vi "SUB_FINDUSB_SND_ID.vi"() -> (3 "Total Sound cards":i32, 4 "PC Sound Card ID":i32, 5 "USB Sound Card ID":i32, 6 "Found USB Snd card":bool)   [LabVIEW 2011]
panel:
  out "Capabilities":T1
  out "Number of Output Devices":i32
  out "Array":string[](array[string])
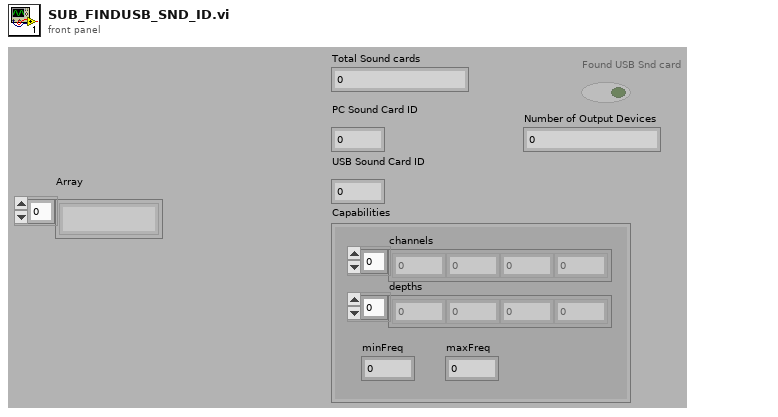
[diagram p1: front panel]
types:
  T1 = cluster{"channels":i32[], "depths":i32[], "minFreq":dbl, "maxFreq":dbl}
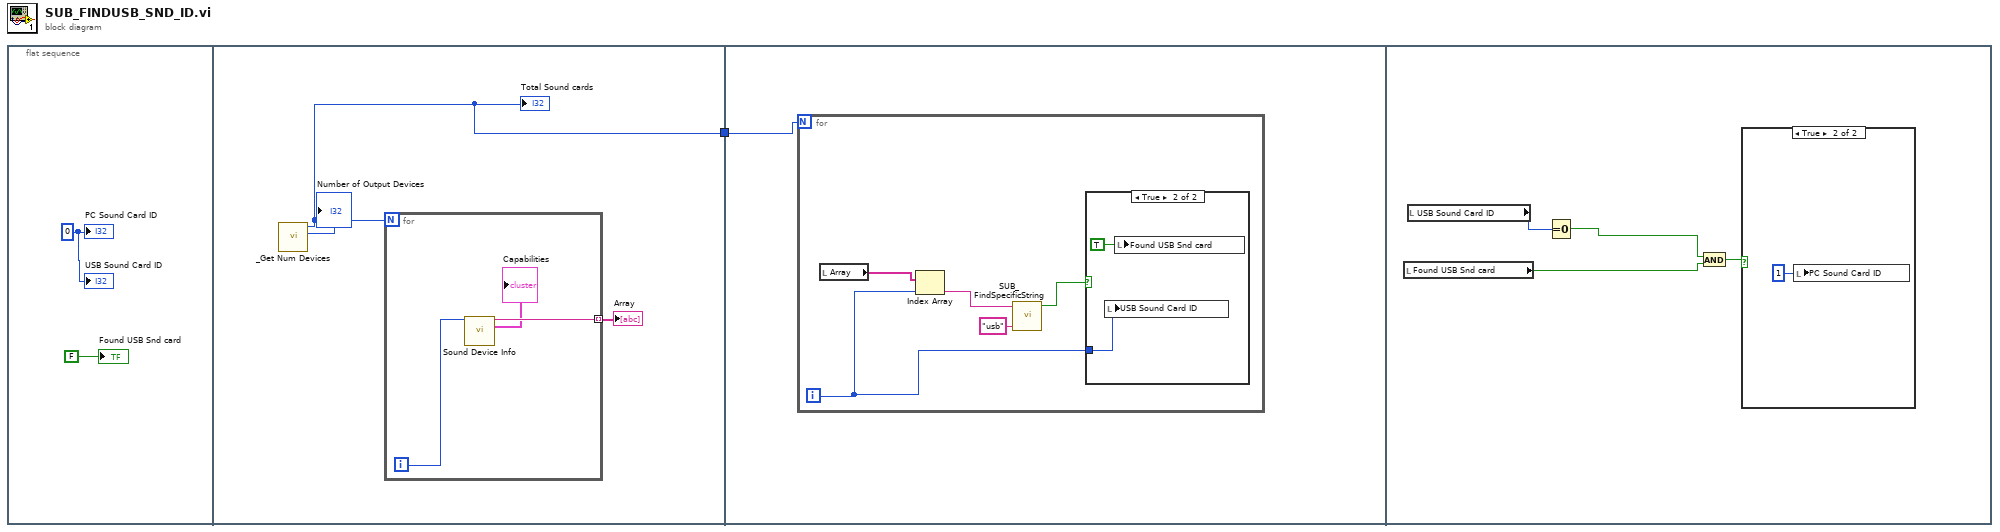
[diagram p0: block diagram]
diagram:
  n1 = flat-sequence {
    tunnel: [w5] -> w1
    tunnel: w1 -> [w10]
    frame #0 {
      w3 = 0
      "PC Sound Card ID" <- w3
      "USB Sound Card ID" <- w3
      "Found USB Snd card" <- FALSE
    }
    frame #1 {
      n2 = call <vilib>:"_Get Num Devices.vi"() -> ("Number of Output Devices"=→"Number of Output Devices":i32, "Number of Input Devices"=w5:i32)  [unwired: 9 in, 1 out]
      "Total Sound cards" <- w5
      n3 = for {
        N: w5 -> [_]
        tunnel: [w8] -> w6 mode=indexing
        i -> [w9]
        n4 = call <vilib>:"Sound Device Info.vi"("device"=w9) -> ("Device Name"=w8:string, "Capabilities"=→"Capabilities":T1)  [unwired: 12 in, 1 out]
      }
      "Array" <- w6
    }
    frame #2 {
      n5 = for {
        N: w10 -> [_]
        i -> [w11]
        n6 = local read "Array"() -> (w15:string[])
        n7 = Index Array(array=w15, index=w11) -> (element=w14:string)
        n8 = call "SUB_FindSpecificString.vi"("Find this String"="usb", "String data"=w14) -> ("Found"=w12:bool)  [unwired: 2 in, 1 out]
        n9 = case shown="True" w12 {
          tunnel: w11 -> [_ w17]
          frame False {
          }
          frame True {
            n10 = local write "USB Sound Card ID"(w17) -> ()
            n11 = local write "Found USB Snd card"(TRUE ("Found USB Snd card")) -> ()
          }
        }
      }
    }
    frame #3 {
      n12 = local read "Found USB Snd card"() -> (w18:bool)
      n13 = local read "USB Sound Card ID"() -> (w21:i32)
      n14 = Equal To 0?(x=w21) -> (x = 0?=w19:bool)
      n15 = And(x=w19, y=w18) -> (x .and. y?=w20:bool)
      n16 = case shown="True" w20 {
        frame False {
        }
        frame True {
          n17 = local write "PC Sound Card ID"(1 ("PC Sound Card ID")) -> ()
        }
      }
    }
  }
